vi "Set Several Test.vi"() -> ()   [LabVIEW 2018, in "AltonTech MALT200817.lvlib"]
doc: "Use this template to build a user interface event handler design pattern. Use this pattern for dialog boxes and other user interfaces. You also can create and execute user-defined events that the VI can handle the same way as user interface events."
uses:
  AltonTech MALT200817.lvlib
panel:
  in  "State Map":u8[](array[numeric])=[255, 255, 255, 255] format="%02x"
  in  "State":bool
  in  "Address":i32=3
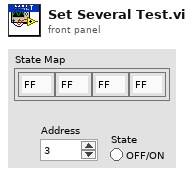
[diagram p1: front panel]
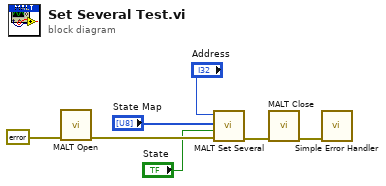
[diagram p0: block diagram]
diagram:
  n1 = call "MALT Open.vi"("error in"=errorcluster {"status"=FALSE, "code"=0, "source"=""}) -> ("error out"=w7:errorcluster)  [unwired: 10 in]
  n2 = call "MALT Set Several.vi"("error in"=w7, "State"="State", "State Map"="State Map", "Address"="Address") -> ("error out"=w2:errorcluster)  [unwired: 7 in]
  n3 = call "MALT Close.vi"("error in"=w2) -> ("error out"=w5:errorcluster)  [unwired: 10 in]
  n4 = call <vilib>:"Simple Error Handler.vi"("error in (no error)"=w5) -> ()  [unwired: 4 in, 5 out]
